vi "uActor_RESERVED.vi"(6 "Original uMsg":refnum<class "uMsg.lvclass">, 8 "error in (no error)":errorcluster, 9 "Data":refnum<class "uData.lvclass">, 10 "Command":string, 11 "uObserver in":refnum<class "uObserver.lvclass">) -> (0 "error out":errorcluster, 1 "reply":refnum<class "uData.lvclass">, 3 "uObserver out":refnum<class "uObserver.lvclass">)   [LabVIEW 2023, in "uLib.lvlib" / "uObserver.lvclass"]
uses:
  uObserver.lvclass
  uData/uData/uData.lvclass
  uMsg/uMsg/uMsg.lvclass
  uObserver.lvclass/uObserver.ctl
  uData/uData/uData.lvclass/uData.ctl
  uMsg/uMsg/uMsg.lvclass/uMsg.ctl
  uData/uData/Condition Tag Name.vi
  uData/uData/Combine Tags.vi
  uTransport/uTransport/uTransport_SendMsg.vi
  uData/uData/Blank Key Reserved String.vi
  uMsg/uMsg/uMsg Update Timestamp.vi
  uTransport/uTransport/uTransport.lvclass
  uActor/uActor.lvclass
  uTransport/uTransport_uActor/uTransport_uActor.lvclass
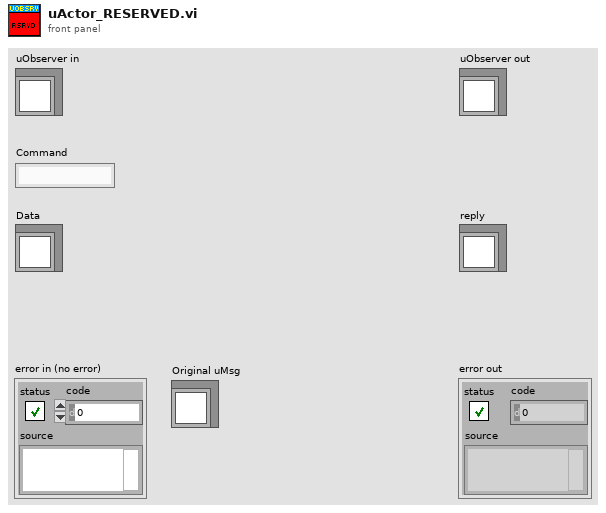
[diagram p1: front panel]
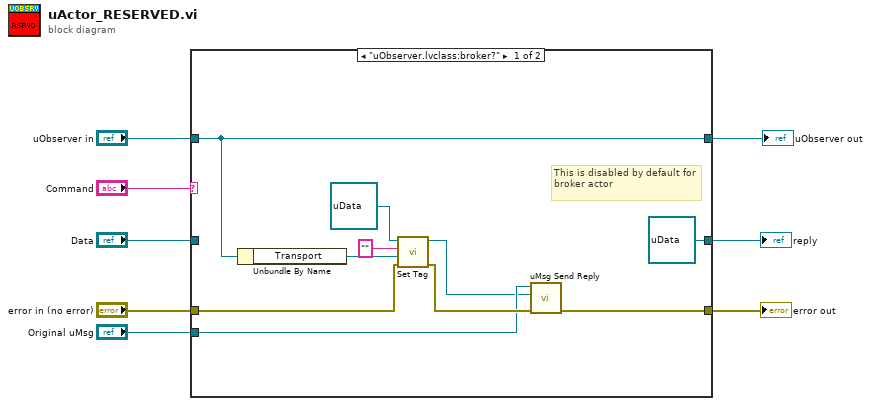
[diagram p0: block diagram]
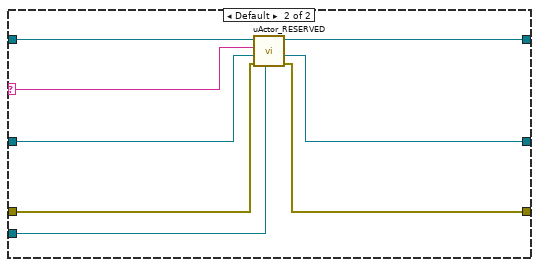
[diagram p2: hidden frame]
diagram:
  n1 = case shown="\"uObserver.lvclass:broker?\"" "Command" {
    selector: "Command" -> [_ w19]
    tunnel: [w11 w24] -> w8
    tunnel: [refnum<class "uData.lvclass"> refnum ("reply") w20] -> w7
    tunnel: [w18 w25] -> w6
    tunnel: "Original uMsg" -> [w10 w22]
    tunnel: "error in (no error)" -> [w15 w23]
    tunnel: "Data" -> [_ w21]
    tunnel: "uObserver in" -> [w18 w26]
    frame "uObserver.lvclass:broker?" {
      # "This is disabled by default for broker actor"
      n2 = Unbundle By Name(w18) -> ("Transport"=w17:refnum<class "uTransport_uActor.lvclass">)
      n3 = call "Set Tag.vi"("error in (no error)"=w15, "Variant"=w17, "tag (case insensitive)"="", "uData in"=refnum<class "uData.lvclass"> refnum) -> ("error out"=w12:errorcluster, "uData out"=w9:refnum<class "uData.lvclass">)  [unwired: 5 in, 1 out]
      n4 = call "uMsg Send Reply.vi"("error in (no error)"=w12, "Reply Data"=w9, "Original Msg"=w10) -> ("error out"=w11:errorcluster)  [unwired: 8 in]
    }
    frame Default {
      n5 = call-parent "uActor_RESERVED.vi"("Original uMsg"=w22, "error in (no error)"=w23, "Data"=w21, "Command"=w19, "uActor in"=w26) -> ("error out"=w24:errorcluster, "reply"=w20:refnum<class "uData.lvclass">, "uActor out"=w25:refnum<class "uObserver.lvclass">)  [unwired: 4 in]
    }
  }
  "error out" <- w8
  "uObserver out" <- w6
  "reply" <- w7
